vi "Lookup API.vi"(7 "API Type":refnum<class "API.lvclass">, 8 "error in (no error)":errorcluster, 10 "Identity":refnum<class "Identity.lvclass">, 11 "Task in":refnum<class "Task.lvclass">) -> (0 "error out":errorcluster, 2 "API":refnum<class "API.lvclass">, 3 "Task out":refnum<class "Task.lvclass">)   [LabVIEW 2020, in "Volatus.lvlib" / "Task.lvclass"]
uses:
  Task.lvclass
  Identity/Identity.lvclass
  API/API.lvclass
  Task.lvclass/Task.ctl
  VolatusAPI/VolatusAPI.lvclass/VolatusAPI.ctl
  Identity/Key.vi
  <vilib>/Utility/error.llb/Error Cluster From Error Code.vi
  VolatusAPI/VolatusAPI.lvclass
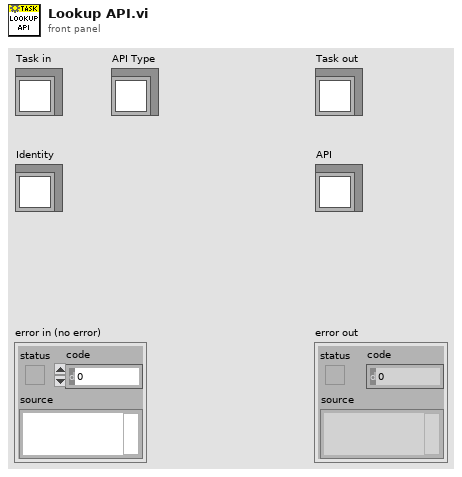
[diagram p1: front panel]
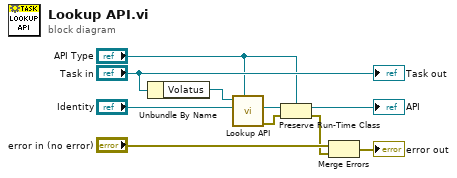
[diagram p0: block diagram]
diagram:
  n1 = Unbundle By Name("Task in") -> ("Volatus"=w8:refnum<class "VolatusAPI.lvclass">)
  n2 = call "Lookup API.vi"("API Type"="API Type", "Identity"="Identity", "VolatusAPI in"=w8) -> ("error out"=w3:errorcluster, "API"=w6:refnum<class "API.lvclass">)  [unwired: 6 in, 1 out]
  n3 = Preserve Run-Time Class(object in=w6, error in=w3, 2:"API Type") -> (object out=→"API":refnum<class "API.lvclass">, error out=w1:errorcluster)
  n4 = Merge Errors("error in (no error)", w1) -> (→"error out":errorcluster)
  "Task out" <- "Task in"
